vi "Wheel Speed Sensor card.vi"(8 "error in (no error)":errorcluster, 11 "Node Ptr":T5 format="%.0x") -> (0 "error out":errorcluster)   [LabVIEW 2014, in "SLSC configuration System Explorer.lvlib"]
uses:
  SLSC configuration System Explorer.lvlib
  <vilib>/NI Veristand/Custom Device API/Custom Device Item Ref.ctl
  Shared/Wheel Speed Sensor Board/WSS Mode Array.ctl
  Shared/Wheel Speed Sensor Board/WSS Mode.ctl
  Type Defs/Card Position.ctl
  Shared/SPI Utility/Slot #.ctl
  Shared/Constants.vi
  <vilib>/NI Veristand/Custom Device API/Get Item Property (U16).vi
  <vilib>/NI Veristand/Custom Device API/Custom Device API.lvlib
  Shared/SLSC configuration Shared.lvlib
panel:
  in  "Card Position":T1 {"Slot #" max=15}
  in  "Header 2":cluster{"Section Name":string}={"Section Name"="Bank 0 Settings"}
  in  "WSS Modes Initial Values":T3
  in  "Header":cluster{"Section Name":string}={"Section Name"="Wheel Speed Sensor Card Settings"}
  in  "Description":string
  in  "Name":string
  # "Channel 1"
  # "Channel 2"
  # "Channel 3"
  # "Channel 4"
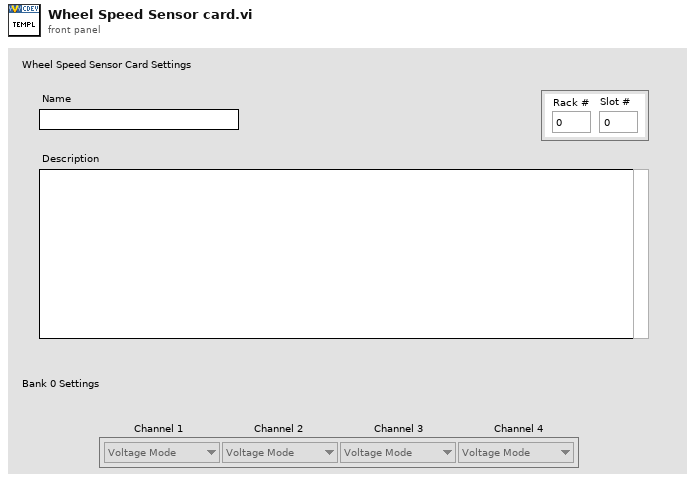
[diagram p1: front panel]
types:
  T1 = typedef "SLSC configuration Shared.lvlib/Card Position.ctl" = cluster{"Rack #":u8, "Slot #":T2}
  T2 = typedef "SLSC configuration Shared.lvlib/Slot #.ctl" = u8
  T3 = typedef "SLSC configuration Shared.lvlib/WSS Mode Array.ctl" = T4[]
  T4 = typedef "SLSC configuration Shared.lvlib/WSS Mode.ctl" = enum8{"Voltage Mode", "Current Mode"}
  T5 = typedef "Custom Device API.lvlib/Custom Device Item Ref.ctl" = u64
  T6 = typedef "Custom Device API.lvlib/Custom Device Item Info.ctl" = cluster{"Name":string, "Is Channel":bool, "GUID":string, "Is Waveform":bool}
  T7 = typedef "Custom Device API.lvlib/Custom Device Commands.ctl" = enum16{"Default", "Item renamed", "Shutdown", "Dynamic button pressed"}
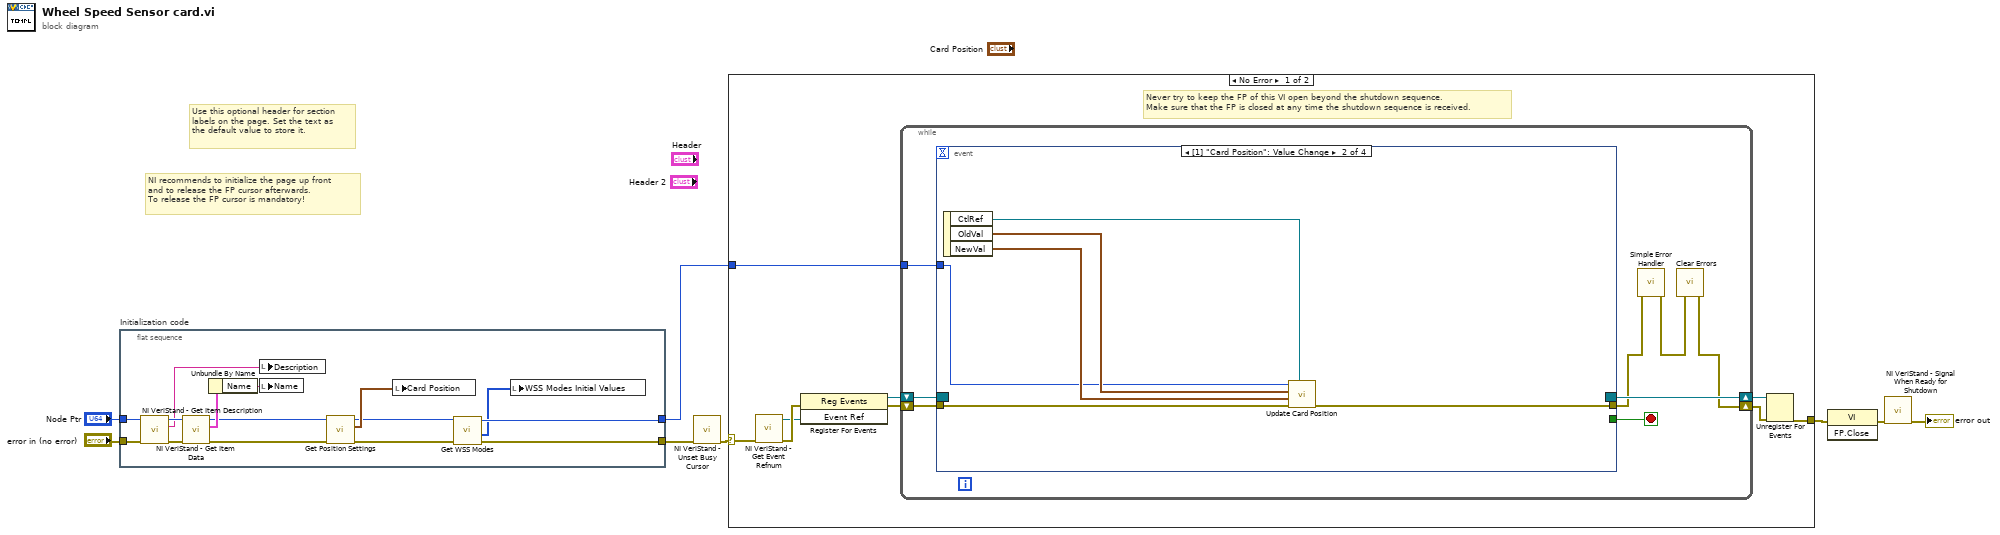
[diagram p0: block diagram]
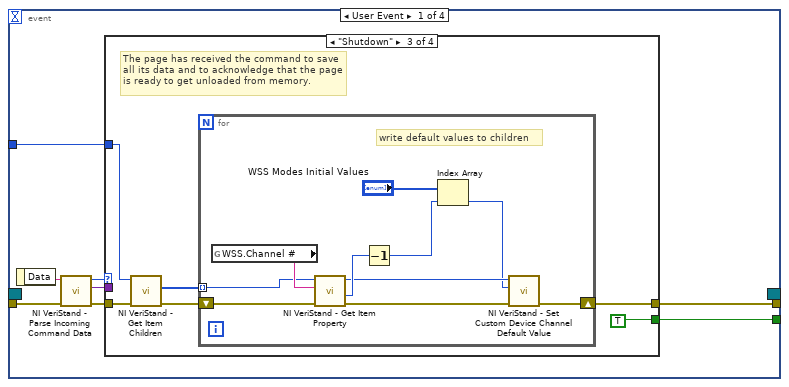
[diagram p2: hidden frame]
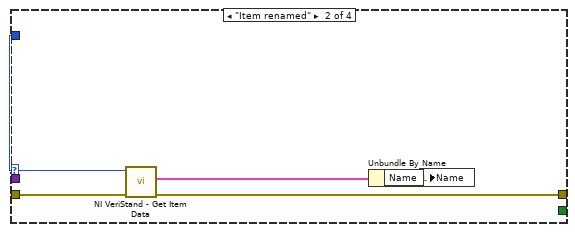
[diagram p4: hidden frame]
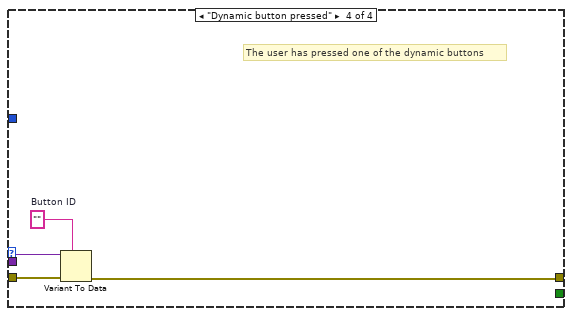
[diagram p5: hidden frame]
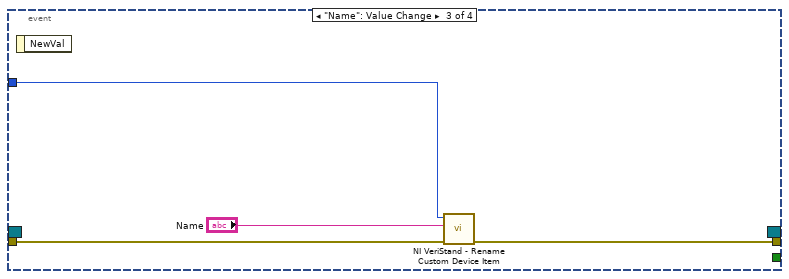
[diagram p6: hidden frame]
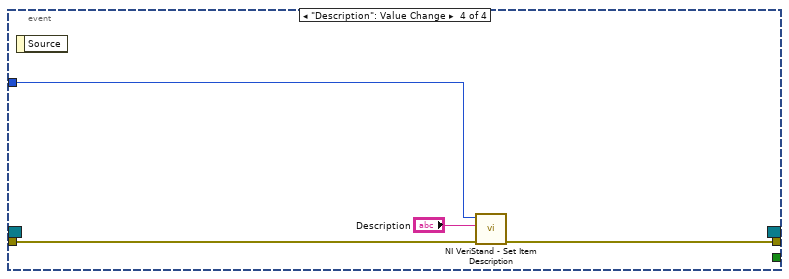
[diagram p7: hidden frame]
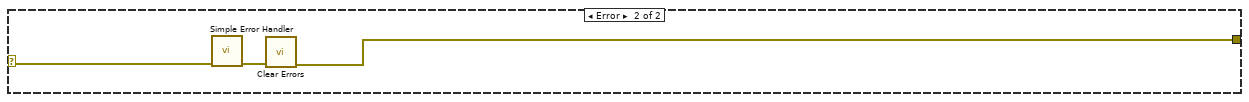
[diagram p8: hidden frame]
diagram:
  # "Use this optional header for section labels on the page. Set the text as the default value to store it."
  # "NI recommends to initialize the page up front\nand to release the FP cursor afterwards.\nTo release the FP cursor is mandatory!"
  n1 = flat-sequence "Initialization code" {
    tunnel: "error in (no error)" -> [w22]
    tunnel: "Node Ptr" -> [w21]
    tunnel: [w11] -> w4
    tunnel: [w12] -> w1
    frame #0 {
      n2 = call <vilib>:"NI VeriStand - Get Item Description.vi"("error in (no error)"=w22, "Item Ref in"=w21) -> ("error out"=w19:errorcluster, "Description"=w20:string, "Item Ref out"=w23:T5)  [unwired: 7 out]
      n3 = call <vilib>:"NI VeriStand - Get Item Data.vi"("error in (no error)"=w19, "Item Ref in"=w23) -> ("error out"=w16:errorcluster, "Item Info"=w18:T6, "Item Ref out"=w15:T5)  [unwired: 7 out]
      n4 = Unbundle By Name(w18) -> ("Name"=w17:string)
      n5 = local write "Description"(w20) -> ()
      n6 = local write "Name"(w17) -> ()
      n7 = call "Get Position Settings.vi"("error in (no error)"=w16, "Item Ref in"=w15) -> ("error out"=w10:errorcluster, "Card Position"=w14:T1, "Item Ref out"=w13:T5)  [unwired: 7 in]
      n8 = local write "Card Position"(w14) -> ()
      n9 = call "Get WSS Modes.vi"("error in (no error)"=w10, "Item Ref in"=w13) -> ("error out"=w11:errorcluster, "Wheel Speed Sensor Modes"=w9:T4[], "Item Ref out"=w12:T5)  [unwired: 6 in, 1 out]
      n10 = local write "WSS Modes Initial Values"(w9) -> ()
    }
  }
  n11 = call <vilib>:"NI VeriStand - Unset Busy Cursor.vi"("error in (no error)"=w4) -> ("error out"=w3:errorcluster)  [unwired: 10 out]
  n12 = case shown="No Error" w3 {
    selector: w3 -> [w24 w91]
    tunnel: [w29 w89] -> w8
    tunnel: w1 -> [w25 _]
    frame No Error {
      # "Never try to keep the FP of this VI open beyond the shutdown sequence.\nMake sure that the FP is closed at any time the shutdown sequence is received."
      n13 = call <vilib>:"NI VeriStand - Get Event Refnum.vi"("error in (no error)"=w24) -> ("error out"=w32:errorcluster, "Event Ref"=w28:refnum<user-event>)  [unwired: 9 out]
      n14 = register-events(error in=w32, w28) -> (reference out=w26:refnum<event-registration>, error out=w27:errorcluster)  [unwired: 1 in]
      n15 = while {
        tunnel: w25 -> [w36]
        shift-right: [w33] -> w30
        shift-left: w27 -> [w39]
        shift-right: [w40] -> w31
        shift-left: w26 -> [w38]
        stop <- w37 stop-if-true
        n16 = event shown="[1] \"Card Position\": Value Change" {
          selector: w38 -> [_ _ _ _]
          dyn-events: [_ _ _ _] -> w40
          timeout: _ -> [_ _ _ _]
          tunnel: w39 -> [w48 w80 w84 w87]
          tunnel: [w44 _ _ _] -> w37
          tunnel: [w43 w79 w83 w86] -> w35
          tunnel: w36 -> [w42 w76 w82 w88]
          event User Event {
            n17 = event-data() -> ("Data"=w47:string)  [unwired: 1 out]
            n18 = call <vilib>:"NI VeriStand - Parse Incoming Command Data.vi"("error in (no error)"=w48, "Incoming data"=w47) -> ("error out"=w46:errorcluster, "Outgoing data"=w41:variant, "Action"=w45:T7)  [unwired: 7 out]
            n19 = case shown="\"Shutdown\"" w45 {
              tunnel: w46 -> [w49 w54 w59 w74]
              tunnel: [_ _ TRUE _] -> w44
              tunnel: [w49 w51 w55 w71] -> w43
              tunnel: w42 -> [_ w53 w58 _]
              tunnel: w41 -> [_ _ _ w73]
              frame "Default", Default {
              }
              frame "Item renamed" {
                n20 = call <vilib>:"NI VeriStand - Get Item Data.vi"("error in (no error)"=w54, "Item Ref in"=w53) -> ("error out"=w51:errorcluster, "Item Info"=w52:T6)  [unwired: 8 out]
                n21 = Unbundle By Name(w52) -> ("Name"=w50:string)
                n22 = local write "Name"(w50) -> ()
              }
              frame "Shutdown" {
                # "The page has received the command to save all its data and to acknowledge that the page is ready to get unloaded from memory."
                n23 = call <vilib>:"NI VeriStand - Get Item Children.vi"("error in (no error)"=w59, "Item Ref in"=w58) -> ("error out"=w57:errorcluster, "Child Refs"=w56:T5[])  [unwired: 6 in, 2 out]
                n24 = for {
                  shift-right: [w61] -> w55
                  shift-left: w57 -> [w69]
                  tunnel: w56 -> [w66] mode=indexing
                  # "write default values to children"
                  n25 = global read "Constants.vi" "WSS.Channel #"() -> (w70:string)
                  n26 = call-poly <vilib>:"NI VeriStand - Get Item Property.vi"("error in (no error)"=w69, "Property Name"=w70, "Item Ref in"=w66) -> ("error out"=w64:errorcluster, "Value"=w67:u16, "Item Ref out"=w63:T5)  [unwired: 5 in, 1 out]
                  n27 = Decrement(x=w67) -> (x-1=w65:u16)
                  n28 = Index Array(array="WSS Modes Initial Values", index=w65) -> (element=w62:T4)
                  n29 = call <vilib>:"NI VeriStand - Set Custom Device Channel Default Value.vi"("error in (no error)"=w64, "Default Value"=w62, "Channel Ref in"=w63) -> ("error out"=w61:errorcluster)  [unwired: 7 in, 1 out]
                }
              }
              frame "Dynamic button pressed" {
                w72 = ""  # Button ID
                # "The user has pressed one of the dynamic buttons"
                n30 = Variant To Data(error in=w74, type=w72, Variant=w73) -> (error out=w71:errorcluster)  [unwired: 1 out]
              }
            }
          }
          event Value Change {
            n31 = event-data() -> ("CtlRef"=w75:refnum<vi>, "OldVal"=w77:T1, "NewVal"=w78:T1)  [unwired: 1 out]
            n32 = call "Update Card Position.vi"("Card Position Ref"=w75, "error in (no error)"=w80, "NewVal"=w78, "OldVal"=w77, "Node Ptr in"=w76) -> ("error out"=w79:errorcluster)  [unwired: 6 in]
          }
          event "Name": Value Change {
            n33 = event-data() -> ()  [unwired: 2 out]
            n34 = call <vilib>:"NI VeriStand - Rename Custom Device Item.vi"("error in (no error)"=w84, "New Name"="Name", "Item Ref in"=w82) -> ("error out"=w83:errorcluster)  [unwired: 1 in, 7 out]
          }
          event "Description": Value Change {
            n35 = event-data() -> ()  [unwired: 2 out]
            n36 = call <vilib>:"NI VeriStand - Set Item Description.vi"("error in (no error)"=w87, "Description"="Description", "Item Ref in"=w88) -> ("error out"=w86:errorcluster)  [unwired: 8 out]
          }
        }
        n37 = call <vilib>:"Simple Error Handler.vi"("error in (no error)"=w35) -> ("error out"=w34:errorcluster)  [unwired: 1 in, 7 out]
        n38 = call <vilib>:"Clear Errors.vi"("error in (no error)"=w34) -> ("error out"=w33:errorcluster)  [unwired: 1 in, 5 out]
      }
      n39 = Unregister For Events(event registration refnum=w31, error in=w30) -> (error out=w29:errorcluster)
    }
    frame Error {
      n40 = call <vilib>:"Simple Error Handler.vi"("error in (no error)"=w91) -> ("error out"=w90:errorcluster)  [unwired: 1 in, 7 out]
      n41 = call <vilib>:"Clear Errors.vi"("error in (no error)"=w90) -> ("error out"=w89:errorcluster)  [unwired: 1 in, 5 out]
    }
  }
  n42 = invoke class="VI" method="FP.Close"(error in=w8) -> (error out=w7:errorcluster)  [unwired: 2 in, 2 out]
  n43 = call <vilib>:"NI VeriStand - Signal When Ready for Shutdown.vi"("error in (no error)"=w7) -> ("error out"=→"error out":errorcluster)  [unwired: 10 out]
